vi "Wait.vi"(8 "error in (no error)":errorcluster, 11 "Simulation in":refnum<class "Simulation.lvclass">) -> (0 "error out":errorcluster, 2 "Ready?":bool, 3 "Simulation out":refnum<class "Simulation.lvclass">)   [LabVIEW 2021, in "Simulation.lvclass"]
uses:
  Simulation.lvclass
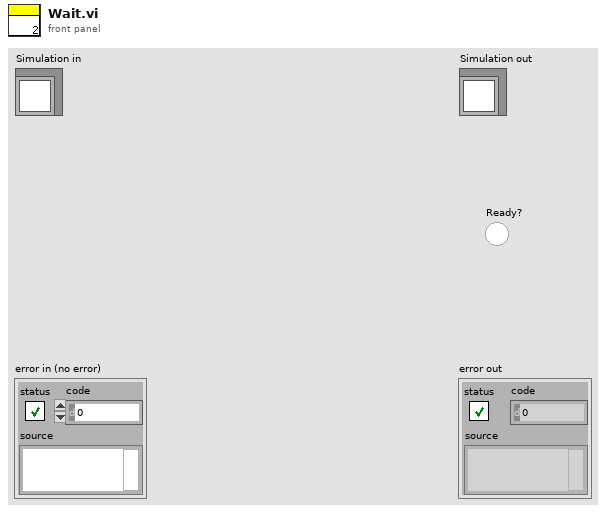
[diagram p1: front panel]
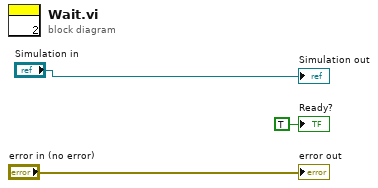
[diagram p0: block diagram]
diagram:
  "error out" <- "error in (no error)"
  "Simulation out" <- "Simulation in"
  "Ready?" <- TRUE ("Ready?")
